vi "Test Compare Float.vi"   [LabVIEW 2020, in "Caraya Test 18.lvlib"]
uses:
  Caraya Test 18.lvlib
  <vilib>/addons/_JKI Toolkits/Caraya/classes/Assert/Assert Equal Value_Variant.vi
  <vilib>/addons/_JKI Toolkits/Caraya/classes/Test/Test.lvclass
  <vilib>/addons/_JKI Toolkits/Caraya/classes/Assert/Assert.lvclass
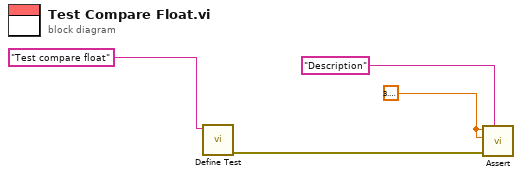
[diagram p0: block diagram]
diagram:
  w3 = 3.141592653589793
  n1 = call <vilib>:"Define Test.vi"("Label (VI Title)"="Test compare float" ("Description")) -> ("error out"=w4:errorcluster)  [unwired: 10 in]
  n2 = call-poly <vilib>:"Assert.vi"("Label"="Description" ("Description"), "error in (no error)"=w4, "Y"=w3, "X"=w3) -> ()  [unwired: 7 in, 1 out]
